vi "Init.vi"(8 "error in":errorcluster, 10 "VIEW":refnum<class "VIEW.lvclass">, 11 "CONTROLLER in":refnum<class "CONTROLLER.lvclass">) -> (0 "error out":errorcluster, 3 "CONTROLLER out":refnum<class "CONTROLLER.lvclass">)   [LabVIEW 2013, in "CONTROLLER.lvclass"]
uses:
  CONTROLLER.lvclass
  View/base/VIEW.lvclass
  CONTROLLER.lvclass/CONTROLLER.ctl
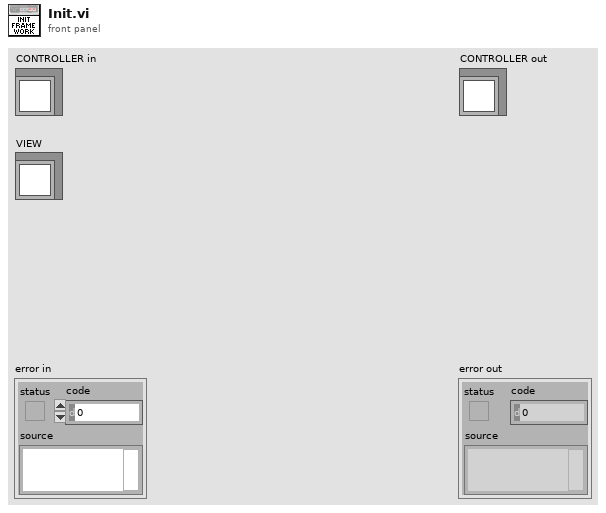
[diagram p1: front panel]
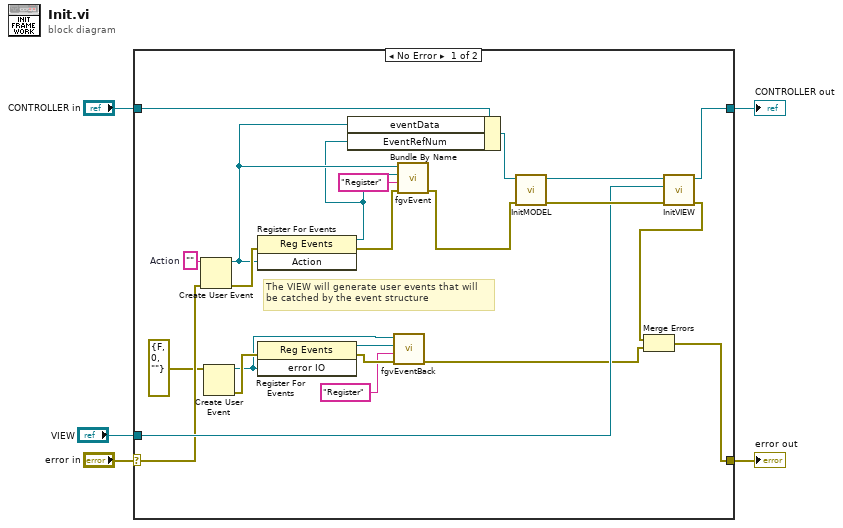
[diagram p0: block diagram]
diagram:
  n1 = case shown="No Error" "error in" {
    selector: "error in" -> [w21 w30]
    tunnel: [w6 w30] -> w4
    tunnel: [w25 w29] -> w2
    tunnel: "CONTROLLER in" -> [w26 w29]
    tunnel: "VIEW" -> [w24 _]
    frame No Error {
      w22 = ""  # Action
      # "The VIEW will generate user events that will\nbe catched by the event structure"
      n2 = Create User Event(user event datatype=w22, error in=w21) -> (user event=w16:refnum<user-event>, error out=w23:errorcluster)
      n3 = Create User Event(user event datatype=errorcluster {"status"=FALSE, "code"=0, "source"=""} ("error IO")) -> (user event=w11:refnum<user-event>, error out=w13:errorcluster)  [unwired: 1 in]
      n4 = register-events(error in=w23, w16) -> (reference out=w15:refnum<event-registration>, error out=w20:errorcluster)  [unwired: 1 in]
      n5 = register-events(error in=w13, w11) -> (reference out=w12:refnum<event-registration>, error out=w10:errorcluster)  [unwired: 1 in]
      n6 = Bundle By Name(cluster=w26, "eventData"=w16, "EventRefNum"=w15) -> (w17:refnum<class "CONTROLLER.lvclass">)
      n7 = call "fgvEventBack.vi"("error in (no error)"=w10, "Cmd"="Register", "EventRefNum"=w12, "EventData"=w11) -> ("error out"=w7:errorcluster)  [unwired: 5 in, 2 out]
      n8 = call "fgvEvent.vi"("error in (no error)"=w20, "Cmd"="Register", "EventRefNum"=w15, "eventData"=w16) -> ("error out"=w19:errorcluster)  [unwired: 5 in, 2 out]
      n9 = call-dynamic "InitMODEL.vi"("error in (no error)"=w19, "CONTROLLER in"=w17) -> ("error out"=w27:errorcluster, "CONTROLLER out"=w28:refnum<class "CONTROLLER.lvclass">)  [unwired: 8 in]
      n10 = call-dynamic "InitVIEW.vi"("error in (no error)"=w27, "VIEW"=w24, "CONTROLLER in"=w28) -> ("error out"=w8:errorcluster, "CONTROLLER out"=w25:refnum<class "CONTROLLER.lvclass">)  [unwired: 7 in]
      n11 = Merge Errors(w8, w7) -> (w6:errorcluster)
    }
    frame Error {
    }
  }
  "error out" <- w4
  "CONTROLLER out" <- w2
